vi "Condense.vi"(1 "Time":dbl format="%<%H:%M:%S>t", 2 "GPIB Address":refnum<visa-resource-name>) -> ()   [LabVIEW 2019]
panel:
  out "Time Remaining":dbl format="%<%H:%M:%S>t"
  in  "stop":bool
  # "He3 Condensing"
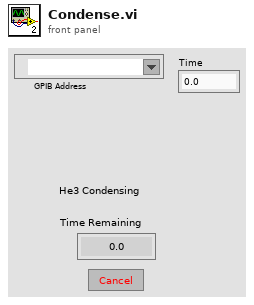
[diagram p1: front panel]
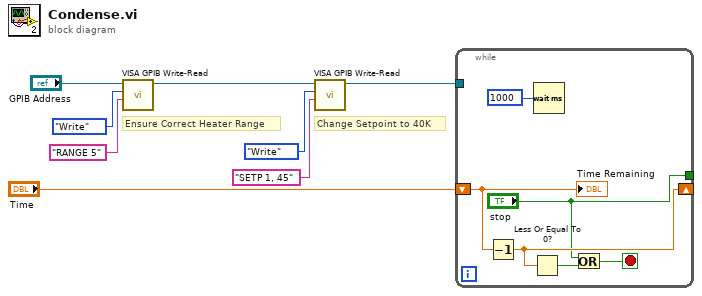
[diagram p0: block diagram]
diagram:
  # "Change Setpoint to 40K"
  # "Ensure Correct Heater Range"
  n1 = call "VISA GPIB Write-Read.vi"("Command"="RANGE 5" ("Command String"), "Action"=enum16{"Write", "Read", "Write & Read"}."Write", "VISA resource name"="GPIB Address") -> ("dup VISA Session"=w7:refnum<visa-resource-name>)  [unwired: 5 in, 3 out]
  n2 = call "VISA GPIB Write-Read.vi"("Command"="SETP 1, 45" ("Command String"), "Action"=enum16{"Write", "Read", "Write & Read"}."Write", "VISA resource name"=w7) -> ("dup VISA Session"=w5:refnum<visa-resource-name>)  [unwired: 5 in, 3 out]
  n3 = while {
    shift-right: [w12] -> _
    shift-left: "Time" -> [w9]
    tunnel: ["stop"] -> _
    tunnel: w5 -> [_]
    stop <- w13 stop-if-true
    n4 = Decrement(x=w9) -> (x-1=w12:dbl)
    n5 = Less Or Equal To 0?(x=w12) -> (x <= 0?=w11:bool)
    n6 = Wait (ms)(milliseconds to wait=u32 1000) -> ()  [unwired: 1 out]
    n7 = Or(x="stop", y=w11) -> (x .or. y?=w13:bool)
    "Time Remaining" <- w9
  }
